vi "creating-a-sub-vi.vi"() -> ()   [LabVIEW 2025]
panel:
  out "Numeric 6":dbl
  out "Numeric 5":dbl
  out "Numeric 4":dbl
  out "Numeric 3":dbl
  in  "Numeric 2":dbl
  in  "Numeric":dbl
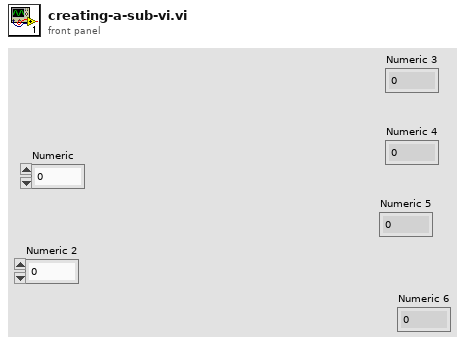
[diagram p1: front panel]
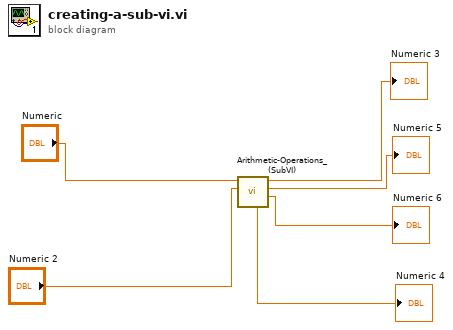
[diagram p0: block diagram]
diagram:
  n1 = call "Arithmetic-Operations_(SubVI).vi"("Numeric 2"="Numeric 2", "Numeric"="Numeric") -> ("Numeric 3"=→"Numeric 6":dbl, "Numeric 4"=→"Numeric 5":dbl, "Numeric 6"=→"Numeric 3":dbl, "Numeric 5"=→"Numeric 4":dbl)  [unwired: 6 in]
